vi "PH_Sixpack_Switch.panel.vi"(0 "object ref":refnum<vi>, 5 "error in (no error)":errorcluster) -> (19 "error out":errorcluster)   [LabVIEW 2014, in "PH_Sixpack_Switch.lvlib"]
doc: "By this VI a hardware switch can be monitored and switched. \n\nThe indicators \"FALSE\", \"TRUE\" and \"SWITCH STATE\" show the value of the Beckhoff-Tag: blue indicates bad tag status reference problems, darkgreen false and lightgreen true. If everything is working fine, \"FALSE\" and \"SWITCH STATE\" should show the same value, while \"TRUE\" has the opposite value. The caption of the sensors for \"FALSE\" and \"TRUE\" are taken out of the database. In case of only one or no sensor these GUI elements are not shown at all.\n\nThe oval button switches. It should be in the same state as the \"SWITCH STATE\" indicator. \n\n\"Delete Instance\" disconnects and removes the instance from the PCS.\n\n\nLicense Agreement for this software:\n\nCopyright (C)\nGesellschaft für Schwerionenforschung, GSI\nPlanckstr. 1\n64291 Darmstadt\nGermany\n\nContact: D.Beck@gsi.de \n\nThis program is free software; you can redistribute it and/or modify it under the terms of the GNU General Public License as published by the Free Software Foundation; either version 2 of the license, or (at your option) any later version.\n\nThis program is distributed in the hope that it will be useful, but WITHOUT ANYW ARRANTY; without even the implied warranty of MERCHANTABILITY or FITNESS FOR A PARTICULAR PURPOSE. See the GNU General License for more details (http://www.gnu.org).\n\nGesellschaft für Schwerionenforschung, GSI\nPlanckstr. 1, 64291 Darmstadt, Germany\nFor all questions and ideas contact: M.Richter@gsi.de, H.Brand@gsi.de or D.Beck@gsi.de.\nLast update: 18-DEC-2002"
uses:
  PH_Sixpack_Switch.lvlib
  PH_Basics/PH_Stepmotor_BaseClass/PH_Stepmotor_BaseClass.Axis Address.ctl
  PH_Basics/PH_Stepmotor_BaseClass/PH_Stepmotor_BaseClass.Axis Settings.ctl
  PH_Basics/PH_Stepmotor_BaseClass/PH_Stepmotor_BaseClass.Motor Type.ctl
  PH_Basics/PH_StatusHandler/PH_StatusHandler.GUI element.ctl
  PH_Basics/PH_Stepmotor_BaseClass/PH_Stepmotor_BaseClass.Axis Direction.ctl
  PH_Basics/PH_Stepmotor_BaseClass/PH_Stepmotor_BaseClass.Axis Activity.ctl
  PH_Basics/PH_AxisGUI_BaseClass/PH_AxisGUI_BaseClass.Axis GUI Refs.ctl
  CS_Core/CSObj/CSObj.lvlib
  PH_Basics/PH_Common/PH_Common.lvlib
  CS_Core/CSSystem/CSSystemLib/CSSystemLib.lvlib
  PH_Basics/PH_AxisGUI_BaseClass/PH_AxisGUI_BaseClass.lvlib
  PH_Basics/PH_Class/PH_Class.lvlib
  PH_Basics/PH_PSDBWriter/PH_PSDBWriter.lvlib
  PH_Basics/PH_StatusHandler/PH_StatusHandler.lvlib
  PH_Basics/PH_Stepmotor_BaseClass/PH_Stepmotor_BaseClass.lvlib
panel:
  out "Status Bar":u32(colorbox)=16777088 caption="Axis1"
  out "Activity":T1
  out "Status":u32(colorbox)=6618880 caption="Axis1"
  in  "StopMotor":bool caption="SetZero"
  in  "Tab Control":enum32{"Move", "Settings", "Info"}(tab)
  in  "Clear Error":bool
  in  "Direction":T2
  in  "Target":string="0" caption="Steps"
  in  "Move":bool
  out "Status":T3 caption="Enabling State"
  in  "Axis_Settings":T4={"Sign change"=FALSE, "Width"=0.0, "Calibration"=0.0, "Unit"="Steps", "Motor Type"=enum."Unspecific", "Unit Width"="", "Unit CF"=""} caption="Axis"
  in  "Reset":bool
  out "Address":T6={"Instance"="N/A", "Motor Nr"=0} caption="Sixpack"
  in  "Set Zero":bool
  out "PSDB Status":u32(colorbox)=6618880 caption="PSDB"
  in  "Exit":bool
  in  "Delete":bool
  # "PCS"
  # "3.40"
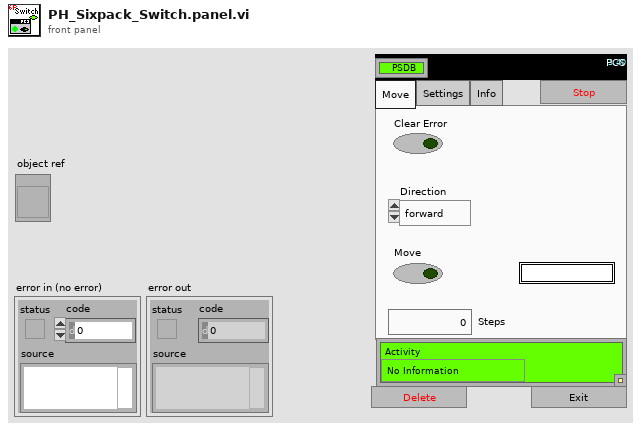
[diagram p1: front panel]
types:
  T1 = typedef "PH_Stepmotor_BaseClass.lvlib/PH_Stepmotor_BaseClass.Axis Activity.ctl" = enum16{"No Information", "stopped", "running", "Failure", "Alarm", "stopped at backward ES", "stopped at foreward ES"}
  T2 = typedef "PH_Stepmotor_BaseClass.lvlib/PH_Stepmotor_BaseClass.Axis Direction.ctl" = enum16{"forward", "backward"}
  T3 = typedef "PH_StatusHandler.lvlib/PH_StatusHandler.GUI element.ctl" = u16
  T4 = typedef "PH_Stepmotor_BaseClass.lvlib/PH_Stepmotor_BaseClass.Axis Settings.ctl" = cluster{"Sign change":bool, "Width":dbl, "Calibration":dbl, "Unit":string, "Motor Type":T5, "Unit Width":string, "Unit CF":string}
  T5 = typedef "PH_Stepmotor_BaseClass.lvlib/PH_Stepmotor_BaseClass.Motor Type.ctl" = enum16{"Unspecific", "OWIS 49.120.2633", "OWIS 49.060.1033", "OWIS 43.040.2558", "Diamond Motion 2200 series", "OWIS 49.120.266B.MV6", "Calorimeter", "Linear Stage 1", "MICOS VT-80", "MICOS VT-80 S", "Standa Rotstage nt0.95A", "PUF RA 320.200", "PUF RA 800.200", "PUF RA 800.400", "PUF RA 400.50", "1324.nn.800.50", "1324.n9c.800.50", "1324.nn.320.200", "1324.nn.400.200", "1324.nn.800.200", "1324.nn.400.50", "1324.8c9c.800.50", "1324.8c9c.400.200"}
  T6 = typedef "PH_Stepmotor_BaseClass.lvlib/PH_Stepmotor_BaseClass.Axis Address.ctl" = cluster{"Instance":string, "Motor Nr":i32}
  T7 = typedef "PH_AxisGUI_BaseClass.lvlib/PH_AxisGUI_BaseClass.Axis GUI Refs.ctl" = cluster{"Back":refnum<vi>, "Forth":refnum<vi>, "Status":refnum<vi>, "Target":refnum<vi>, "Address":refnum<vi>, "Status Bar":refnum<vi>, "Settings":refnum<vi>, "Activity":refnum<vi>, "Clear Error":refnum<vi>}
  T8 = typedef "PH_AxisGUI_BaseClass.lvlib/PH_AxisGUI_BaseClass.i attribute.ctl" = cluster{"Axes":T9[]}
  T9 = typedef "PH_AxisGUI_BaseClass.lvlib/PH_AxisGUI_BaseClass.Axis Attributes.ctl" = cluster{"Axis GUI Refs":T7, "Address":T6, "Name":string, "Label \"Back\"":string, "Labell \"Forth\"":string, "Moving?":bool}
  T10 = typedef "PH_Sixpack_Switch.lvlib/PH_Sixpack_Switch.i attribute.ctl" = cluster{"GUI Refs":cluster{"Delete":refnum<vi>, "Move":refnum<vi>, "Direction":refnum<vi>}, "remote controlled?":bool, "Move":bool, "Direction":T2}
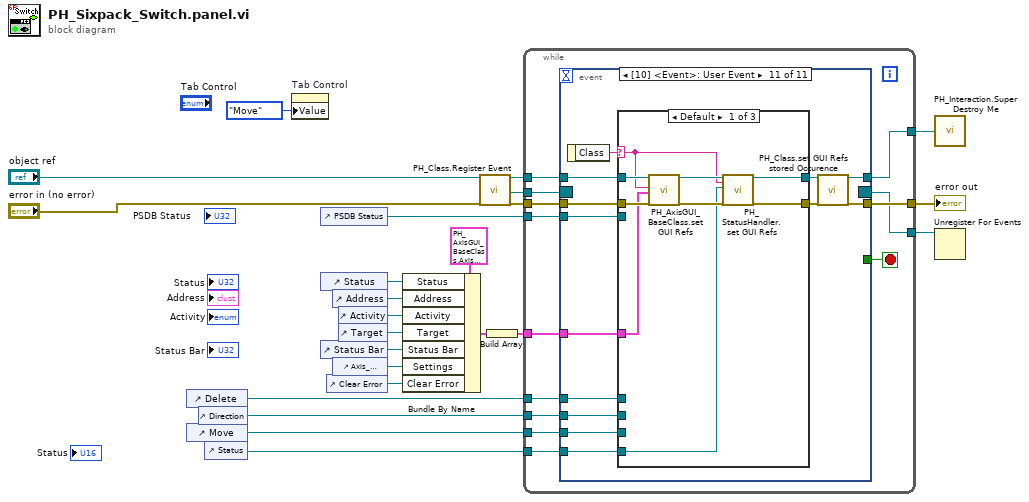
[diagram p0: block diagram]
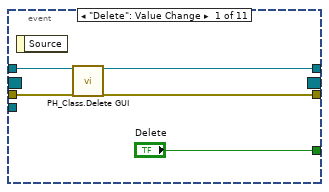
[diagram p2: hidden frame]
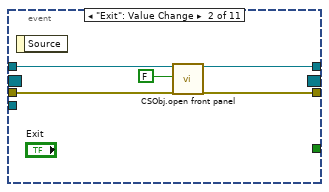
[diagram p3: hidden frame]
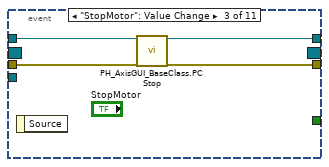
[diagram p4: hidden frame]
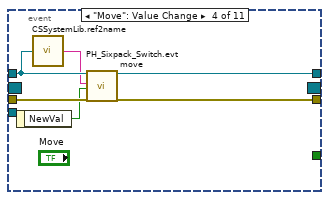
[diagram p5: hidden frame]
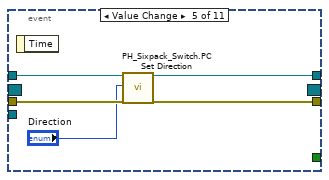
[diagram p6: hidden frame]
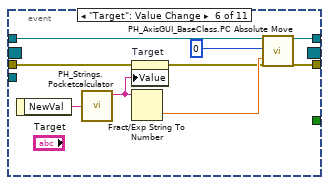
[diagram p7: hidden frame]
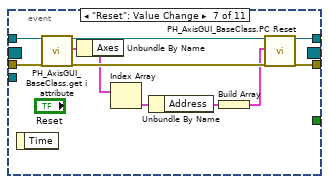
[diagram p8: hidden frame]
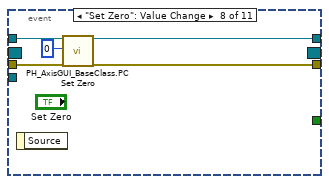
[diagram p9: hidden frame]
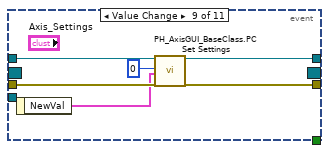
[diagram p10: hidden frame]
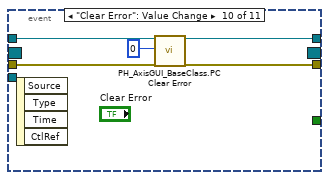
[diagram p11: hidden frame]
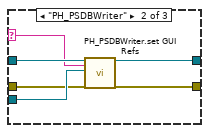
[diagram p12: hidden frame]
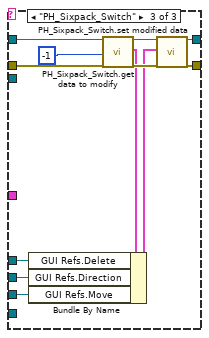
[diagram p13: hidden frame]
diagram:
  n1 = control-ref of="Delete"() -> (w8:refnum<vi>)
  n2 = control-ref of="Move"() -> (w6:refnum<vi>)
  n3 = control-ref of="Direction"() -> (w7:refnum<vi>)
  n4 = control-ref of="Status"() -> (w1:refnum<vi>)
  n5 = property on="Tab Control" class="TabCtl (strict)"("Value"=enum32{"Move", "Settings", "Info"}."Move" ("Tab Control")) -> ()  [unwired: 2 in, 2 out]
  n6 = control-ref of="PSDB Status"() -> (w4:refnum<vi>)
  n7 = control-ref of="Status"() -> (w14:refnum<vi>)
  n8 = control-ref of="Status Bar"() -> (w16:refnum<vi>)
  n9 = control-ref of="Clear Error"() -> (w13:refnum<vi>)
  n10 = control-ref of="Address"() -> (w20:refnum<vi>)
  n11 = control-ref of="Axis_Settings"() -> (w18:refnum<vi>)
  n12 = control-ref of="Activity"() -> (w15:refnum<vi>)
  n13 = control-ref of="Target"() -> (w19:refnum<vi>)
  n14 = Bundle By Name(cluster=T7 {"Back"=refnum, "Forth"=refnum, "Status"=refnum, "Target"=refnum, "Address"=refnum, "Status Bar"=refnum, "Settings"=refnum, "Activity"=refnum, "Clear Error"=refnum} ("GUI Refs"), "Status"=w14, "Address"=w20, "Activity"=w15, "Target"=w19, "Status Bar"=w16, "Settings"=w18, "Clear Error"=w13) -> (w21:T7)
  n15 = call "PH_Class.Register Event.vi"("i ref in"="object ref", "error in (no error)"="error in (no error)") -> ("i ref out"=w11:refnum<vi>, "Event Registration Refnum"=w10:refnum<event-registration>, "error out"=w12:errorcluster)  [unwired: 15 in]
  n16 = Build Array(w21) -> (w5:T7[])
  n17 = while {
    tunnel: w11 -> [w34]
    tunnel: [w33] -> w24
    tunnel: w12 -> [w36]
    tunnel: [w35] -> w23
    tunnel: w10 -> [w32]
    tunnel: [w31] -> w9
    tunnel: w8 -> [w30]
    tunnel: w1 -> [w29]
    tunnel: w7 -> [w28]
    tunnel: w6 -> [w27]
    tunnel: w5 -> [w26]
    tunnel: w4 -> [w25]
    stop <- w37 stop-if-true
    n18 = event shown="[10] <Event>: User Event" {
      selector: w32 -> [_ _ _ _ _ _ _ _ _ _ _]
      dyn-events: [_ _ _ _ _ _ _ _ _ _ _] -> w31
      timeout: _ -> [_ _ _ _ _ _ _ _ _ _ _]
      tunnel: ["Delete" _ _ _ _ _ _ _ _ _ _] -> w37
      tunnel: w34 -> [w41 w46 w49 w54 w62 w68 w75 w86 w92 w97 w110]
      tunnel: w36 -> [w40 w45 w48 w57 w61 w65 w74 w84 w90 w95 w105]
      tunnel: [w39 w44 w50 w55 w59 w69 w72 w83 w89 w94 w101] -> w35
      tunnel: [w38 w43 w51 w56 w60 w67 w73 w85 w91 w96 w99] -> w33
      tunnel: w30 -> [_ _ _ _ _ _ _ _ _ _ w109]
      tunnel: w29 -> [_ _ _ _ _ _ _ _ _ _ w108]
      tunnel: w28 -> [_ _ _ _ _ _ _ _ _ _ w107]
      tunnel: w27 -> [_ _ _ _ _ _ _ _ _ _ w106]
      tunnel: w26 -> [_ _ _ _ _ _ _ _ _ _ w103]
      tunnel: w25 -> [_ _ _ _ _ _ _ _ _ _ w102]
      event "Delete": Value Change {
        n19 = event-data() -> ()  [unwired: 1 in, 1 out]
        n20 = call "PH_Class.Delete GUI.vi"("VI in"=w41, "error in (no error)"=w40) -> ("VI out"=w38:refnum<vi>, "error out"=w39:errorcluster)  [unwired: 16 in]
      }
      event "Exit": Value Change {
        n21 = event-data() -> ()  [unwired: 1 in, 1 out]
        n22 = call "CSObj.open front panel.vi"("i ref in"=w46, "frontPanelOpen"=FALSE ("front panel open"), "error in (no error)"=w45) -> ("i ref out"=w43:refnum<vi>, "error out"=w44:errorcluster)  [unwired: 15 in]
      }
      event "StopMotor": Value Change {
        n23 = event-data() -> ()  [unwired: 1 in, 1 out]
        n24 = call "PH_AxisGUI_BaseClass.PC Stop.vi"("VI in"=w49, "error in (no error)"=w48) -> ("VI out"=w51:refnum<vi>, "error out"=w50:errorcluster)  [unwired: 16 in]
      }
      event "Move": Value Change {
        n25 = event-data() -> ("NewVal"=w52:bool)  [unwired: 1 in]
        n26 = call "CSSystemLib.ref2name.vi"("obj refnum"=w54) -> ("name"=w53:string)
        n27 = call "PH_Sixpack_Switch.evt move.vi"("i ref in"=w54, "Instance"=w53, "Move"=w52, "error in (no error)"=w57) -> ("i ref out"=w56:refnum<vi>, "error out"=w55:errorcluster)  [unwired: 14 in]
      }
      event Value Change {
        n28 = event-data() -> ()  [unwired: 1 in, 1 out]
        n29 = call "PH_Sixpack_Switch.PC Set Direction.vi"("i ref in"=w62, "Direction"="Direction", "error IO"=w61) -> ("i ref out"=w60:refnum<vi>, "error out"=w59:errorcluster)  [unwired: 15 in]
      }
      event "Target": Value Change {
        n30 = event-data() -> ("NewVal"=w66:string)  [unwired: 1 in]
        n31 = call "PH_Strings.Pocketcalculator.vi"("Input"=w66) -> ("String Double"=w63:string)  [unwired: 3 out]
        n32 = property on="Target" class="Str"(error in=w65, "Value"=w63) -> (error out=w64:errorcluster)  [unwired: 1 in, 1 out]
        n33 = Fract/Exp String To Number(string=w63) -> (number=w71:dbl)  [unwired: 3 in, 1 out]
        n34 = call "PH_AxisGUI_BaseClass.PC Absolute Move.vi"("i ref in"=w68, "Axis"=0, "Position [Units]"=w71, "error in"=w64) -> ("i ref out"=w67:refnum<vi>, "error out"=w69:errorcluster)  [unwired: 14 in]
      }
      event "Reset": Value Change {
        n35 = event-data() -> ()  [unwired: 1 in, 1 out]
        n36 = call "PH_AxisGUI_BaseClass.get i attribute.vi"("i ref in"=w75, "error in (no error)"=w74) -> ("i ref out"=w82:refnum<vi>, "i attribute"=w80:T8, "error out"=w81:errorcluster)  [unwired: 15 in]
        n37 = Unbundle By Name(w80) -> ("Axes"=w78:T9[])
        n38 = Index Array(array=w78) -> (element=w79:T9)  [unwired: 1 in]
        n39 = Unbundle By Name(w79) -> ("Address"=w77:T6)
        n40 = Build Array(w77) -> (w76:T6[])
        n41 = call "PH_AxisGUI_BaseClass.PC Reset.vi"("i ref in"=w82, "Addresses"=w76, "error in"=w81) -> ("i ref out"=w73:refnum<vi>, "error out"=w72:errorcluster)  [unwired: 15 in]
      }
      event "Set Zero": Value Change {
        n42 = event-data() -> ()  [unwired: 1 in, 1 out]
        n43 = call "PH_AxisGUI_BaseClass.PC Set Zero.vi"("VI in"=w86, "Axis"=0, "error in (no error)"=w84) -> ("VI out"=w85:refnum<vi>, "error out"=w83:errorcluster)  [unwired: 15 in]
      }
      event Value Change {
        n44 = event-data() -> ("NewVal"=w88:T4)  [unwired: 1 in]
        n45 = call "PH_AxisGUI_BaseClass.PC Set Settings.vi"("VI in"=w92, "Axis"=0, "NewVal"=w88, "error in (no error)"=w90) -> ("VI out"=w91:refnum<vi>, "error out"=w89:errorcluster)  [unwired: 14 in]
      }
      event "Clear Error": Value Change {
        n46 = event-data() -> ()  [unwired: 1 in, 4 out]
        n47 = call "PH_AxisGUI_BaseClass.PC Clear Error.vi"("i ref in"=w97, "Axis"=0, "error in"=w95) -> ("i ref out"=w96:refnum<vi>, "error out"=w94:errorcluster)  [unwired: 15 in]
      }
      event User Event {
        n48 = event-data() -> ("Class"=w111:string)  [unwired: 1 in]
        n49 = case shown="Default" w111 {
          selector: w111 -> [w113 w121 _]
          tunnel: w110 -> [w120 w126 w135]
          tunnel: [w114 w123 w134] -> w100
          tunnel: w109 -> [_ _ w133]
          tunnel: w108 -> [w112 _ _]
          tunnel: w107 -> [_ _ w130]
          tunnel: w106 -> [_ _ w129]
          tunnel: w105 -> [w119 w124 w128]
          tunnel: [w116 w122 w127] -> w104
          tunnel: w103 -> [w117 _ _]
          tunnel: w102 -> [_ w125 _]
          frame Default {
            n50 = call "PH_AxisGUI_BaseClass.set GUI Refs.vi"("i ref in"=w120, "Class"=w113, "Axis GUI Base Class Refs"=w117, "error in"=w119) -> ("i ref out"=w115:refnum<vi>, "error out"=w118:errorcluster)  [unwired: 14 in]
            n51 = call "PH_StatusHandler.set GUI Refs.vi"("i ref in"=w115, "Class"=w113, "GUI Ref"=w112, "error in (no error)"=w118) -> ("i ref out"=w114:refnum<vi>, "error out"=w116:errorcluster)  [unwired: 14 in]
          }
          frame "PH_PSDBWriter" {
            n52 = call "PH_PSDBWriter.set GUI Refs.vi"("i ref in"=w126, "Class"=w121, "Ref PSDB Status"=w125, "error in"=w124) -> ("i ref out"=w123:refnum<vi>, "error out"=w122:errorcluster)  [unwired: 14 in]
          }
          frame "PH_Sixpack_Switch" {
            n53 = call "PH_Sixpack_Switch.get data to modify.vi"("i ref in"=w135, "ms timeout (10000)"=-1, "error in (no error)"=w128) -> ("i ref out"=w138:refnum<vi>, "i attribute"=w132:T10, "error out"=w137:errorcluster)  [unwired: 13 in, 1 out]
            n54 = Bundle By Name(cluster=w132, "GUI Refs.Delete"=w133, "GUI Refs.Direction"=w130, "GUI Refs.Move"=w129) -> (w131:T10)
            n55 = call "PH_Sixpack_Switch.set modified data.vi"("i ref in"=w138, "i attribute"=w131, "error in (no error)"=w137) -> ("i ref out"=w134:refnum<vi>, "error out"=w127:errorcluster)  [unwired: 15 in]
          }
        }
        n56 = call "PH_Class.set GUI Refs stored Occurence.vi"("i ref in"=w100, "error in (no error)"=w104) -> ("i ref out"=w99:refnum<vi>, "error out"=w101:errorcluster)  [unwired: 16 in]
      }
    }
  }
  "error out" <- w23
  n57 = call "PH_Interaction.Super Destroy Me.vi"("i ref out"=w24) -> ()
  n58 = Unregister For Events(event registration refnum=w9) -> ()  [unwired: 1 in, 1 out]
